vi "client.vi"(7 "httpRequestID":u32) -> ()   [LabVIEW 2011]
doc: "This VI is a state machine that can be ran from a Browser."
uses:
  server/database/Users/User Record.ctl
  <vilib>/wsapi/NI_WebServices.lvlib
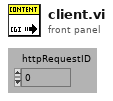
[diagram p1: front panel]
types:
  T1 = typedef "User Record.ctl" = cluster{"ixUser":i32, "sxUsername":string, "sLastName":string, "sFirstName":string, "sEmail":string, "sPassword":string, "tLoginTime":timestamp, "sLoginComputer":string, "fAdministrator":bool, "fRunSequences":bool, "fModifySequences":bool, "fRunScenarios":bool, "fModifyScenarios":bool, "fModifyTemplates":bool, "fModifyUsers":bool, "fModifyStations":bool, "fModifyFields":bool}
  T2 = typedef "Connection Refnum.ctl" = cluster{"Environment Handle":i32, "Connection Handle":i32}
  T3 = typedef "Keyed Array.ctl" = cluster{"keys":string[], "values":string[]}
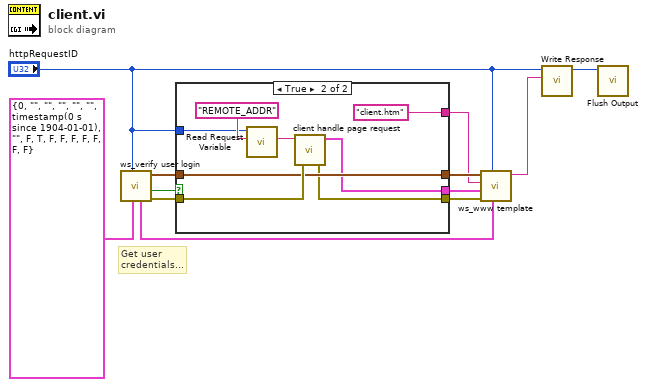
[diagram p0: block diagram]
diagram:
  # "Get user \ncredentials..."
  n1 = call "ws_verify user login.vi"("Required Permisions"=T1 {"ixUser"=0, "sxUsername"="", "sLastName"="", "sFirstName"="", "sEmail"="", "sPassword"="", "tLoginTime"=timestamp(0 s since 1904-01-01), "sLoginComputer"="", "fAdministrator"=FALSE, "fRunSequences"=TRUE, "fModifySequences"=FALSE, "fRunScenarios"=FALSE, "fModifyScenarios"=FALSE, "fModifyTemplates"=FALSE, "fModifyUsers"=FALSE, "fModifyStations"=FALSE, "fModifyFields"=FALSE} ("User Record"), "httpRequestID"="httpRequestID") -> ("error out"=w12:errorcluster, "User Verified\nand Spartan\nAuthorized?"=w10:bool, "DB Connection Ref"=w11:T2, "User"=w6:T1)  [unwired: 6 in]
  n2 = case shown="True" w10 {
    tunnel: [w13 w18] -> w7
    tunnel: w12 -> [w13 w20]
    tunnel: w11 -> [w14 w19]
    tunnel: [w14 w19] -> w8
    tunnel: [_ "client.htm" ("Template (\"\")")] -> w4
    tunnel: [_ w16] -> w5
    tunnel: "httpRequestID" -> [_ w15]
    frame False {
    }
    frame True {
      n3 = call <vilib>:"Read Request Variable.vi"("variable name"="REMOTE_ADDR" ("key"), "httpRequestID"=w15) -> ("value"=w21:string)  [unwired: 7 in, 2 out]
      n4 = call "client handle page request.vi"("error in (no error)"=w20, "Client IP (\"\")"=w21) -> ("error out"=w18:errorcluster, "Template Keys"=w16:T3)  [unwired: 4 out]
    }
  }
  n5 = call "ws_www template.vi"("User"=w6, "httpRequestID"="httpRequestID", "error in (no error)"=w7, "Template Keys (empty)"=w5, "Template (\"\")"=w4, "DB Connection Ref"=w8) -> ("HTTP Template Content"=w1:string)  [unwired: 5 in]
  n6 = call <vilib>:"Write Response.vi"("response string"=w1, "httpRequestID"="httpRequestID") -> ("httpRequestID out"=w3:u32)  [unwired: 8 in, 1 out]
  n7 = call <vilib>:"Flush Output.vi"("httpRequestID"=w3) -> ()  [unwired: 9 in, 2 out]
